vi "北斗配置同步 (子VI).vi"   [LabVIEW 2016, in "环境动力监测库.lvlib" / "NMEA.lvlib"]
uses:
  NMEA.lvlib
  <vilib>/Utility/config.llb/NI_LVConfig.lvlib
types:
  T1 = cluster{"监测项描述:输出":string, "连接方式":enum16{"串口", "TCP"}, "端口":string, "IP address:":string, "Port:":string, "站号":u64, "传感器型号":string, "波特率":u64, "data bits":u64, "停止位":u16, "奇偶校验":u16, "声光告警启用":bool}
  T2 = typedef "NI_LVConfig.lvlib/Config Data RefNum.ctl" = refnum<k1>
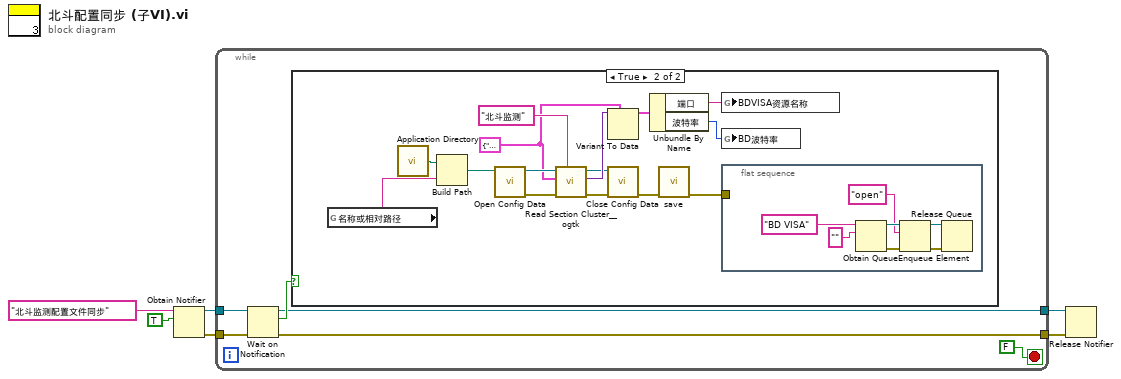
[diagram p0: block diagram]
diagram:
  n1 = Obtain Notifier(name (unnamed)="北斗监测配置文件同步" ("名称（未命名）"), notification data type=TRUE) -> (notifier out=w3:refnum<notifier>, error out=w4:errorcluster)  [unwired: 2 in, 1 out]
  n2 = while {
    tunnel: w3 -> [w12]
    tunnel: w4 -> [w11]
    tunnel: [w8] -> w5
    tunnel: [w7] -> w6
    stop <- FALSE stop-if-true
    n3 = Wait on Notification(notifier=w12, error in (no error)=w11) -> (notifier out=w8:refnum<notifier>, notification=w10:bool, error out=w7:errorcluster)  [unwired: 2 in, 1 out]
    n4 = case shown="True" w10 {
      frame False {
      }
      frame True {
        w14 = T1 {"监测项描述:输出"="", "连接方式"=enum."串口", "端口"="", "IP address:"="", "Port:"="", "站号"=19200, "传感器型号"="", "波特率"=19200, "data bits"=8, "停止位"=10, "奇偶校验"=0, "声光告警启用"=FALSE} ("输出簇")
        n5 = global read "内部交互全局变量.vi" "名称或相对路径"() -> (w13:string)
        n6 = call <vilib>:"Application Directory.vi"() -> ("Application Directory"=w22:path)
        n7 = Build Path(base path=w22, name or relative path=w13) -> (appended path=w21:path)
        n8 = call <vilib>:"Open Config Data.vi"("configuration file path"=w21) -> ("error out"=w20:errorcluster, "refnum"=w19:T2)  [unwired: 8 in, 1 out]
        n9 = call <userlib>:"Read Section Cluster__ogtk.vi"("section (optional)"="北斗监测", "error in (no error)"=w20, "Section Formatted Cluster Type"=w14, "refnum"=w19) -> ("error out"=w25:errorcluster, "Section Formatted Cluster"=w26:variant, "dup refnum"=w24:T2)  [unwired: 3 in, 2 out]
        n10 = Variant To Data(type=w14, Variant=w26) -> (data=w27:T1)  [unwired: 1 in, 1 out]
        n11 = call <vilib>:"Close Config Data.vi"("error in (no error)"=w25, "refnum"=w24) -> ("error out"=w16:errorcluster)  [unwired: 8 in, 1 out]
        n12 = Unbundle By Name(w27) -> ("端口"=w18:string, "波特率"=w17:u64)
        n13 = call "save.vi"("error in (no error)"=w16) -> ("error out"=w15:errorcluster)  [unwired: 10 in]
        n14 = global write "断电保存全局变量.vi" "BDVISA资源名称"(w18) -> ()
        n15 = global write "断电保存全局变量.vi" "BD波特率"(w17) -> ()
        n16 = flat-sequence {
          tunnel: w15 -> [_]
          frame #0 {
            n17 = Obtain Queue(name (unnamed)="BD VISA" ("名称（未命名）"), element data type="") -> (queue out=w33:refnum<queue>, error out=w32:errorcluster)  [unwired: 3 in, 1 out]
            n18 = Enqueue Element(queue=w33, element="open", error in (no error)=w32) -> (queue out=w30:refnum<queue>, error out=w29:errorcluster)  [unwired: 1 in, 1 out]
            n19 = Release Queue(queue=w30, error in (no error)=w29) -> ()  [unwired: 1 in, 3 out]
          }
        }
      }
    }
  }
  n20 = Release Notifier(notifier=w5, error in (no error)=w6) -> ()  [unwired: 1 in, 3 out]
